vi "LVDimInterface.dis_add_service.vi"(1 "serviceName":string, 2 "typeDescriptor":string, 3 "data":string, 5 "error in (no error)":errorcluster, 7 "safeMode":bool=TRUE) -> (14 "my_serviceID":i32, 19 "error out":errorcluster)   [LabVIEW 2014, in "LVDimInterface.lvlib"]
doc: "Add a service to a DIM server. Use \"update service\" to publish new data. If no longer used, a service should be removed using \"remove service\". \n\nImportant: One must call \"start serving\" to declare the new service to the dim name server.\n\nHistory: 16-DEC-2005, Dietrich Beck\n\nCopyright (C)\nGesellschaft für Schwerionenforschung, GSI\nPlanckstr. 1\n64291 Darmstadt\nGermany\n\nContact: D.Beck@gsi.de \n\nThis program is free software; you can redistribute it and/or modify it under the terms of the \nGNU General Public License as published by the Free Software Foundation; either version 2 of the license, or (at your option) any later version.\n\nThis program is distributed in the hope that it will be useful, but WITHOUT ANY WARRANTY; without even the implied warranty of MERCHANTABILITY or FITNESS FOR A PARTICULAR PURPOSE. See the GNU General License for more details (http://www.gnu.org).\n\nGesellschaft für Schwerionenforschung, GSI\nPlanckstr. 1, 64291 Darmstadt, Germany\nFor all questions and ideas contact D. Beck.\nLast update: 16-DEC-2005"
uses:
  LVDimInterface.lvlib
  <vilib>/NI/syslog/_subVIs/TypeDefs/syslog_severity_codes.ctl
  bin/libDimWrapper.dll
  bin/libDimWrapper.so
  bin/libDimWrapperSPL.dll
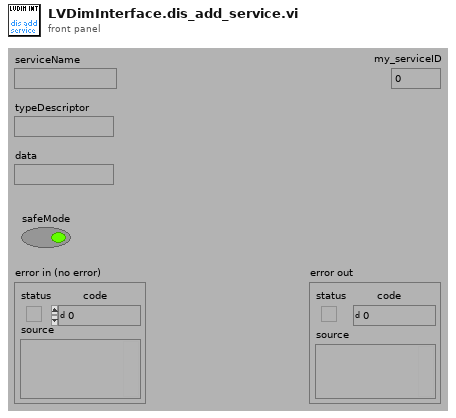
[diagram p1: front panel]
types:
  T1 = typedef "syslog_severity_codes.ctl" = enum16{"emergency", "alert", "critical", "error", "warning", "notice", "info", "debug"}
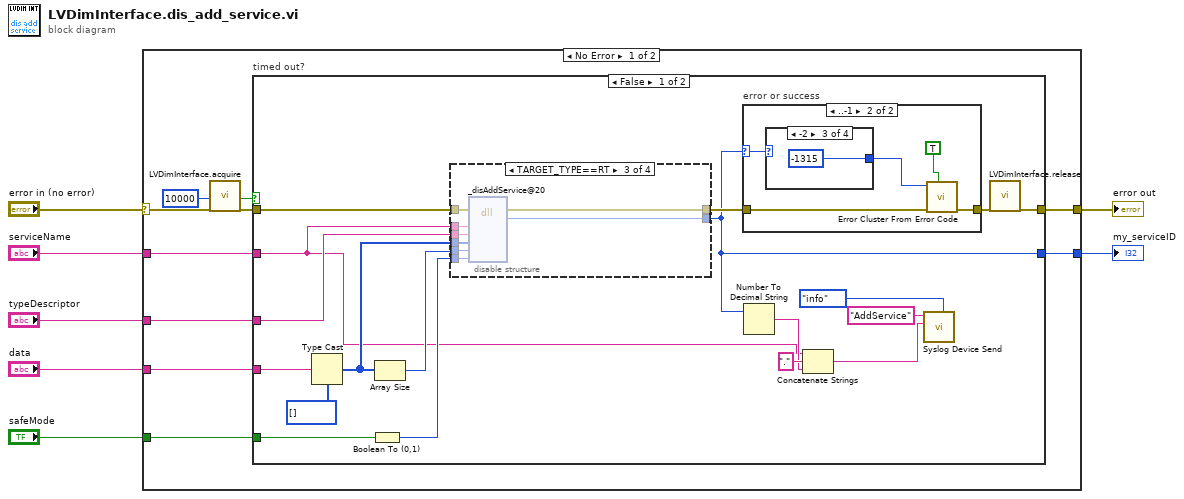
[diagram p0: block diagram]
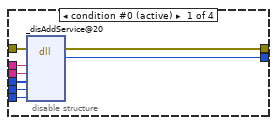
[diagram p2: hidden frame]
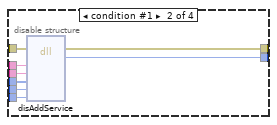
[diagram p3: hidden frame]
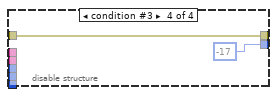
[diagram p4: hidden frame]
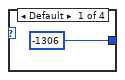
[diagram p6: hidden frame]
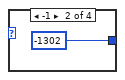
[diagram p7: hidden frame]
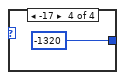
[diagram p8: hidden frame]
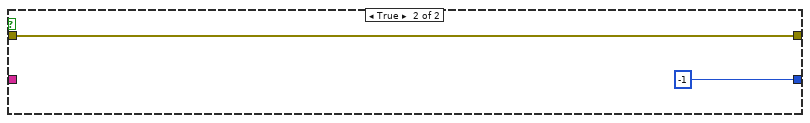
[diagram p9: hidden frame]
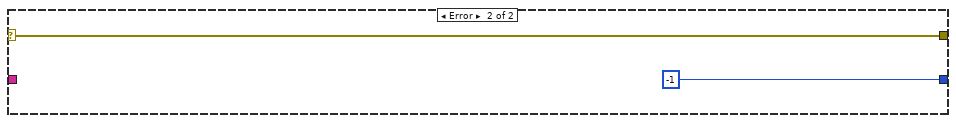
[diagram p10: hidden frame]
diagram:
  n1 = case shown="No Error" "error in (no error)" {
    selector: "error in (no error)" -> [w9 w74]
    tunnel: "serviceName" -> [w17 _]
    tunnel: "data" -> [w14 _]
    tunnel: [w16 -1 ("my_serviceID")] -> w5
    tunnel: [w8 w74] -> w3
    tunnel: "typeDescriptor" -> [w15 _]
    tunnel: "safeMode" -> [w13 _]
    frame No Error {
      n2 = call "LVDimInterface.acquire.vi"("ms timeout (10000)"=10000 ("ms timeout (-1)"), "error in (no error)"=w9) -> ("timed out"=w10:bool, "error out"=w12:errorcluster)  [unwired: 16 in]
      n3 = case "timed out?" shown="False" w10 {
        tunnel: w17 -> [w18 _]
        tunnel: [w20 -1 ("my_serviceID")] -> w16
        tunnel: w15 -> [w35 _]
        tunnel: w14 -> [w33 _]
        tunnel: w13 -> [w30 _]
        tunnel: w12 -> [w28 w72]
        tunnel: [w25 w72] -> w8
        frame False {
          n4 = Type Cast(type=i8[] [], x=w33) -> (*(type *) &x=w32:i8[])
          n5 = Boolean To (0,1)(Boolean=w30) -> (0, 1=w29:i16)
          n6 = Array Size(array=w32) -> (size(s)=w34:i32)
          n7 = disable-structure "Conditional Disable Structure" shown="TARGET_TYPE==RT" {
            disable-tunnel: w18 -> [w43 w51 w59 _]
            disable-tunnel: [w42 w50 w58 -17 ("my_serviceID")] -> w20
            disable-tunnel: w35 -> [w41 w49 w57 _]
            disable-tunnel: w34 -> [w40 w48 w56 _]
            disable-tunnel: w32 -> [w39 w47 w55 _]
            disable-tunnel: w29 -> [w38 w46 w54 _]
            disable-tunnel: w28 -> [w37 w45 w53 w60]
            disable-tunnel: [w36 w44 w52 w60] -> w27
            frame condition #0 (active) {
              n8 = dll-call lib="D:/Git/PHELIX-framework/CSlibraries-extern/DimLVEvent/bin/libDimWrapper.dll" fn="_disAddService@20" label="disAddService"(error in=w37, "serviceName"=w43, "typeDescriptor"=w41, "data"=w39, "size"=w40, "safeMode"=w38) -> (error out=w36:errorcluster, "my_serviceID"=w42:i32)  [unwired: 7 in, 1 out]
            }
            frame condition #1 {
              n9 = dll-call lib="D:/Git/CS-framework/CSlibraries/DimLVEvent/bin/libDimWrapper.so" fn="disAddService"(error in=w45, "serviceName"=w51, "typeDescriptor"=w49, "data"=w47, "size"=w48, "safeMode"=w46) -> (error out=w44:errorcluster, "my_serviceID"=w50:i32)  [unwired: 7 in, 1 out]
            }
            frame condition #2 {
              n10 = dll-call lib="D:/Git/CS-framework/CSlibraries/DimLVEvent/bin/libDimWrapperSPL.dll" fn="_disAddService@20" label="libDimWrapper.so:disAddService"(error in=w53, "serviceName"=w59, "typeDescriptor"=w57, "data"=w55, "size"=w56, "safeMode"=w54) -> (error out=w52:errorcluster, "my_serviceID"=w58:i32)  [unwired: 7 in, 1 out]
            }
            frame condition #3 {
            }
          }
          n11 = case "error or success" shown="..-1" w20 {
            selector: w20 -> [_ w67]
            tunnel: w27 -> [w62 w66]
            tunnel: [w62 w65] -> w26
            frame 0, Default {
            }
            frame ..-1 {
              n12 = case shown="-2" w67 {
                tunnel: [-1306 ("f") -1302 ("code") -1315 ("code") -1320 ("code")] -> w64
                frame Default {
                }
                frame -1 {
                }
                frame -2 {
                }
                frame -17 {
                }
              }
              n13 = call <vilib>:"Error Cluster From Error Code.vi"("show call chain? (False)"=TRUE ("status"), "error in (no error)"=w66, "error code (0)"=w64) -> ("error out"=w65:errorcluster)  [unwired: 6 in]
            }
          }
          n14 = Number To Decimal String(number=w20) -> (decimal integer string=w21:string)  [unwired: 1 in]
          n15 = Concatenate Strings(w18, "." ("string"), w21) -> (w19:string)
          n16 = call <vilib>:"Syslog Device Send.vi"("Severity Code (error)"=syslog_severity_codes."info", "Message Content"=w19, "Message Tag"="AddService") -> ()  [unwired: 7 in, 2 out]
          n17 = call "LVDimInterface.release.vi"("error in (no error)"=w26) -> ("error out"=w25:errorcluster)  [unwired: 18 in]
        }
        frame True {
        }
      }
    }
    frame Error {
    }
  }
  "error out" <- w3
  "my_serviceID" <- w5
